vi "get method name.vi"(8 "error in (no error)":errorcluster, 11 "Request in":variant) -> (0 "error out":errorcluster, 2 "Name":string, 3 "Request out":variant)   [LabVIEW 2017, in "JSONRPC Server.lvclass"]
uses:
  JSONRPC Server.lvclass
  <vilib>/National Instruments/Variant Data Manipulation/Variant Data Manipulation.lvlib
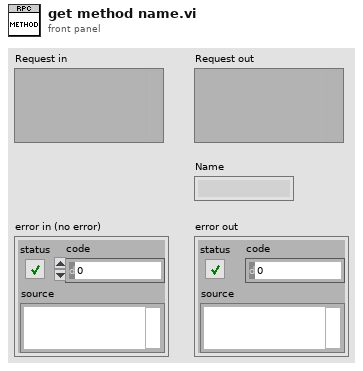
[diagram p1: front panel]
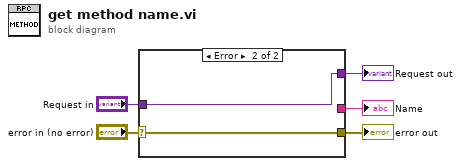
[diagram p0: block diagram]
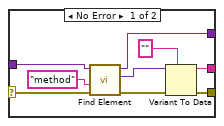
[diagram p2: hidden frame]
diagram:
  n1 = case shown="Error" "error in (no error)" {
    selector: "error in (no error)" -> [w6 w15]
    tunnel: [w13 w16] -> w5
    tunnel: [w12 w15] -> w4
    tunnel: [w11 _] -> w3
    tunnel: "Request in" -> [w7 w16]
    frame No Error {
      n2 = call <vilib>:"Find Element.vi"("error in (no error)"=w6, "Name"="method", "Variant (Cluster) in"=w7) -> ("error out"=w9:errorcluster, "element"=w14:variant, "Variant (Cluster) out"=w13:variant)  [unwired: 4 in, 2 out]
      n3 = Variant To Data(error in=w9, type="" ("Name"), Variant=w14) -> (data=w11:string, error out=w12:errorcluster)
    }
    frame Error {
    }
  }
  "Request out" <- w5
  "error out" <- w4
  "Name" <- w3
